vi "Defaults Operator.vi"(7 "Operation (Load)":enum16{"Load", "Save"}(ring), 8 "error in (no error)":errorcluster, 10 "INI's path":path, 11 "VI's path":path) -> (0 "error out":errorcluster, 2 "INI's path":path, 3 "VI's path":path)   [LabVIEW 2020, in "Save-Load-Defaults.lvlib"]
uses:
  Save-Load-Defaults.lvlib
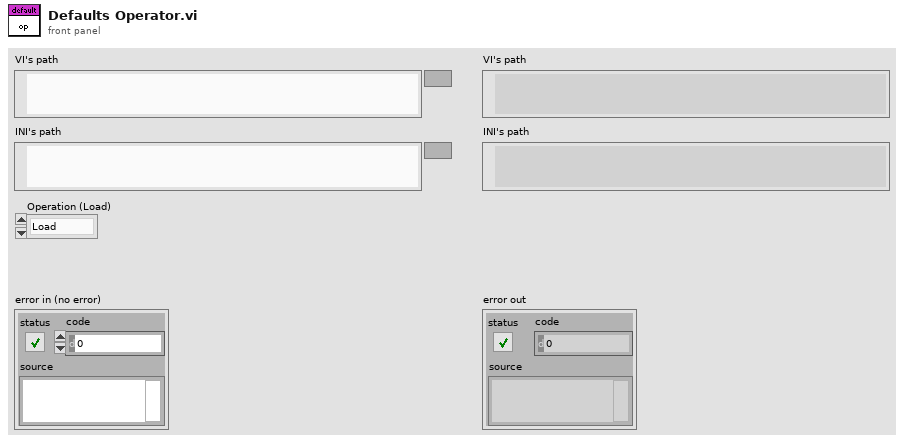
[diagram p1: front panel]
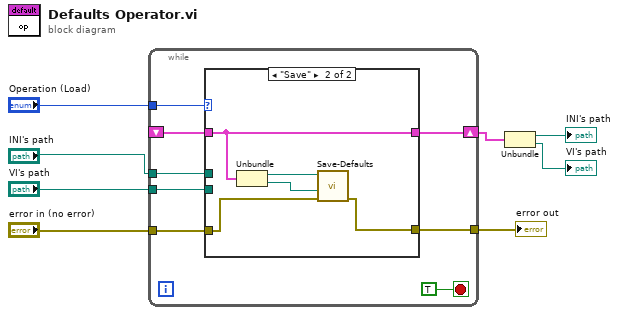
[diagram p0: block diagram]
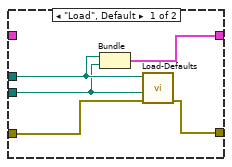
[diagram p2: hidden frame]
diagram:
  n1 = while {
    shift-right: [w10] -> w3
    shift-left: _ -> [w9]
    tunnel: "Operation (Load)" -> [w15]
    tunnel: "VI's path" -> [w14]
    tunnel: "INI's path" -> [w13]
    tunnel: "error in (no error)" -> [w12]
    tunnel: [w11] -> w6
    stop <- TRUE stop-if-true
    n2 = case shown="\"Save\"" w15 {
      tunnel: w14 -> [w18 _]
      tunnel: w13 -> [w19 _]
      tunnel: w12 -> [w21 w26]
      tunnel: [w20 w25] -> w11
      tunnel: [w17 w22] -> w10
      tunnel: w9 -> [_ w22]
      frame "Load", Default {
        n3 = Bundle("INI's path"=w19, "VI's path"=w18) -> (w17:cluster{"INI's path":path, "VI's path":path})  [unwired: 1 in]
        n4 = call "Load-Defaults.vi"("error in (no error)"=w21, "VI path"=w18, "configuration file path"=w19) -> ("error out"=w20:errorcluster)  [unwired: 8 in]
      }
      frame "Save" {
        n5 = Unbundle(w22) -> ("INI's path"=w24:path, "VI's path"=w23:path)
        n6 = call "Save-Defaults.vi"("error in (no error)"=w26, "VI path"=w23, "configuration file path"=w24) -> ("error out"=w25:errorcluster)  [unwired: 8 in]
      }
    }
  }
  "error out" <- w6
  n7 = Unbundle(w3) -> ("INI's path"=→"INI's path":path, "VI's path"=→"VI's path":path)
